vi "PolySetIcon.vi"   [LabVIEW 2020]
types:
  T1 = cluster{"VIPath":path, "Menu Name":string, "Selector Name":string}[]
  T2 = typedef "imagedata.ctl" = cluster{"image type":i32, "image depth":i32, "image":u8[], "mask":u8[], "colors":u32[], "Rectangle":cluster{"left":i16, "top":i16, "right":i16, "bottom":i16}}
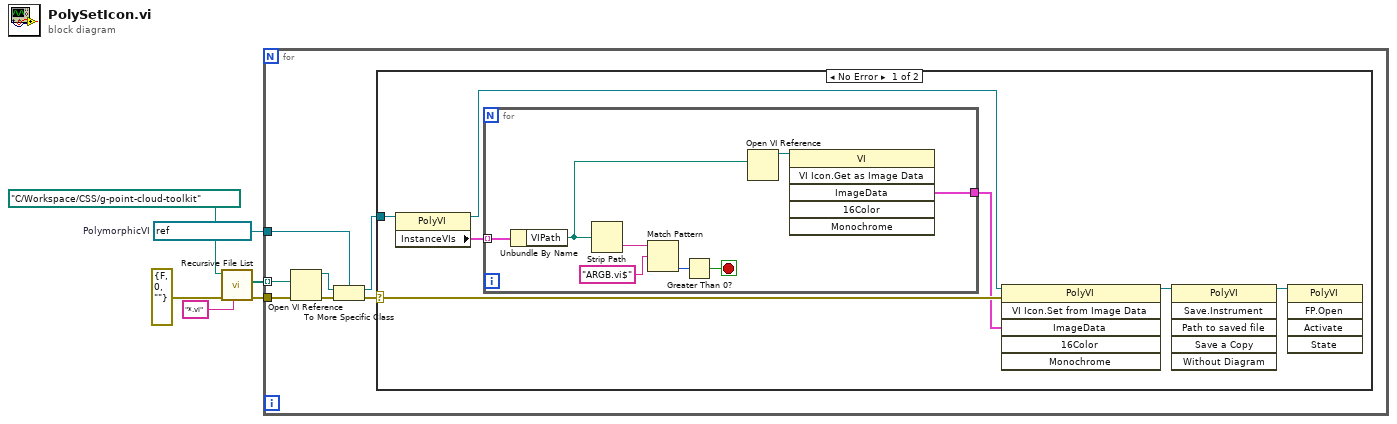
[diagram p0: block diagram]
diagram:
  w3 = refnum<vi> refnum  # PolymorphicVI
  n1 = call <vilib>:"Recursive File List.vi"("pattern"="*.vi", "error in (no error)"=errorcluster {"status"=FALSE, "code"=0, "source"=""} ("error out"), "Folder Path"=path "C:/Workspace/CSS/g-point-cloud-toolkit") -> ("error out"=w6:errorcluster, "All Files in Dir"=w5:path[])  [unwired: 4 in, 3 out]
  n2 = for {
    tunnel: w6 -> [w13]
    tunnel: w5 -> [w12] mode=indexing
    tunnel: w3 -> [w11]
    n3 = Open VI Reference(vi path=w12, error in (no error)=w13) -> (vi reference=w10:refnum<vi>, error out=w9:errorcluster)  [unwired: 4 in]
    n4 = To More Specific Class(target class=w11, reference=w10, error in=w9) -> (specific class reference=w7:refnum<vi>, error out=w8:errorcluster)
    n5 = case shown="No Error" w8 {
      selector: w8 -> [w20 _]
      tunnel: w7 -> [w19 _]
      frame No Error {
        n6 = property class="PolyVI"(reference=w19) -> (reference out=w18:refnum<vi>, "InstanceVIs"=w17:T1)  [unwired: 1 in, 1 out]
        n7 = for {
          tunnel: w17 -> [w28] mode=indexing
          tunnel: [w23] -> w16
          stop <- w22 stop-if-true
          n8 = Unbundle By Name(w28) -> ("VIPath"=w24:path)
          n9 = Strip Path(path=w24) -> (name=w27:string)  [unwired: 1 out]
          n10 = Match Pattern(string=w27, regular expression="ARGB.vi$") -> (offset past match=w25:i32)  [unwired: 1 in, 3 out]
          n11 = Greater Than 0?(x=w25) -> (x > 0?=w22:bool)
          n12 = Open VI Reference(vi path=w24) -> (vi reference=w21:refnum<vi>)  [unwired: 5 in, 1 out]
          n13 = invoke class="VI" method="VI Icon.Get as Image Data"(reference=w21) -> ("ImageData"=w23:T2)  [unwired: 5 in, 5 out]
        }
        n14 = invoke class="PolyVI" method="VI Icon.Set from Image Data"(reference=w18, error in=w20, "ImageData"=w16) -> (reference out=w15:refnum<vi>)  [unwired: 3 in, 5 out]
        n15 = invoke class="PolyVI" method="Save.Instrument"(reference=w15) -> (reference out=w14:refnum<vi>)  [unwired: 5 in, 5 out]
        n16 = invoke class="PolyVI" method="FP.Open"(reference=w14) -> ()  [unwired: 4 in, 5 out]
      }
      frame Error {
      }
    }
  }
